vi "1A TemperatureLogger.vi"() -> ()   [LabVIEW 2011]
doc: "Elizabeth Mahon\n\nThis takes the data from the cRIO's built-in temperature sensor and saves it to a CSV file.\nPretty simple - talks to the FPGA to get the data, then sends it to a CSV file."
uses:
  <vilib>/Platform/storage/Storage.llb/usiOverwriteOptions.ctl
  <vilib>/Platform/storage/Storage.llb/usiSequenceRepresentation.ctl
  <vilib>/FPGAPlugInAG/cRIO-9113/niLvFpga_Open_cRIO-9113.vi
  <vilib>/rvi/interface/common/dynamic/niFpgaDynamicAddResources.vi
  <vilib>/Utility/error.llb/Error Cluster From Error Code.vi
  <vilib>/rvi/errors/niLvFpgaAdjustHostInterfaceError.vi
  <vilib>/FPGAPlugInAG/Dynamic/niLvFpga_Close_Dynamic.vi
  <vilib>/Platform/storage/lvStorage.llb/_openStorageWithRootAutoDetect.vi
  <vilib>/Platform/storage/lvStorage.llb/xStorage/xStorageSupp/ErrorOut.vi
  <vilib>/Platform/storage/lvStorage.llb/_createOrGetExplicitChildObject.vi
  <vilib>/Platform/storage/lvStorage.llb/_createOrGetByNameExplicitChildObject.vi
  <vilib>/Platform/storage/lvStorage.llb/_saveInt16Channel.vi
  <vilib>/Platform/storage/Storage.llb/Get Object Info.vi
  <vilib>/Platform/storage/Storage.llb/__closeStorageFromObject.vi
  <vilib>/rvi/interface/nirviOpenFPGA/nirviOpenFPGA.xnode
  FPGA Bitfiles/SailBot_FPGATarget_1ATemperatureRea_2D2CF993.lvbitx
  FPGA/1A Temperature Reader.vi
  <vilib>/rvi/interface/nirviMethod/nirviMethod.xnode
  <vilib>/rvi/interface/nirviCloseFPGA/nirviCloseFPGA.xnode
  <vilib>/Platform/storage/lvStorage.llb/xStorage/Open Data Storage/Open Data Storage.xnode
  <vilib>/Platform/storage/lvStorage.llb/xStorage/Write Data/Write Data.xnode
  <vilib>/Platform/storage/lvStorage.llb/xStorage/Close Data Storage/Close Data Storage.xnode
  <vilib>/FPGAPlugInAG/Dynamic/niLvFpga_ReadFifo_Dynamic.vi
  <vilib>/rvi/errors/niLvFpgaMergeErrorWithErrorCode.vi
panel:
  out "Temperature Data":i16[](graph)
  in  "stop":bool
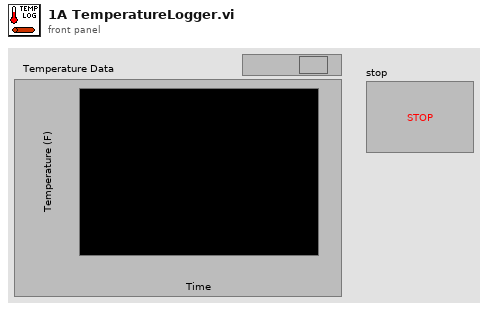
[diagram p1: front panel]
types:
  T1 = enum16{"open", "open or create", "create or replace", "create", "open (read only)"}
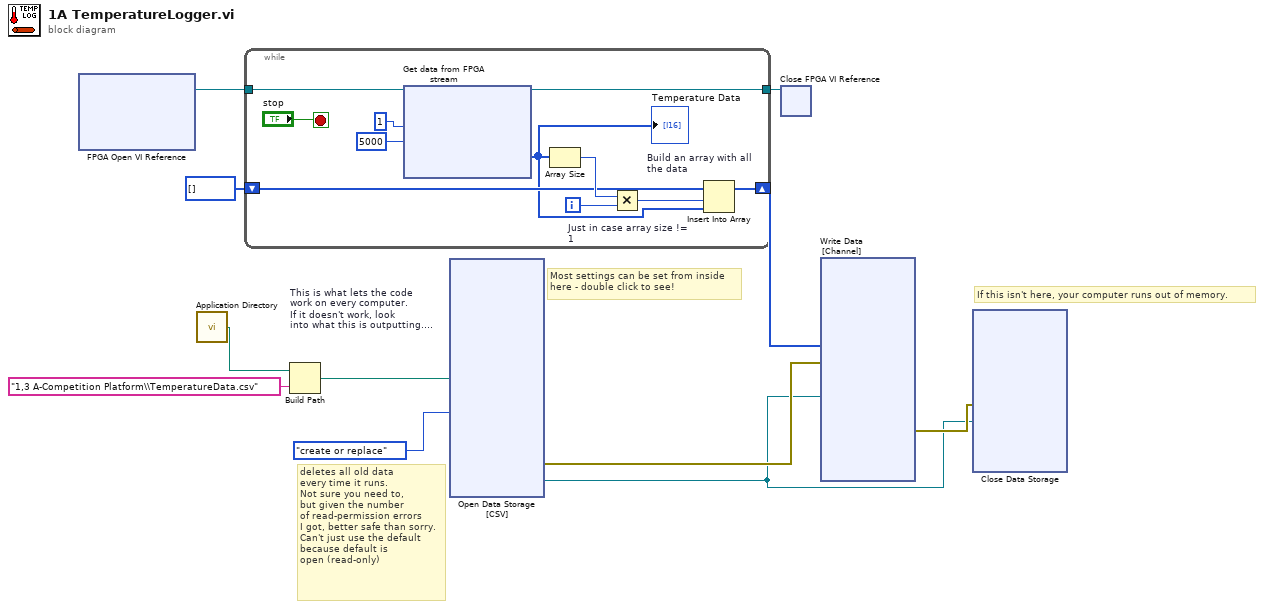
[diagram p0: block diagram]
diagram:
  # "Most settings can be set from inside\nhere - double click to see!"
  # "If this isn't here, your computer runs out of memory."
  # "deletes all old data\nevery time it runs.\nNot sure you need to,\nbut given the number\nof read-permission errors\nI got, better safe than sorry.\nCan't just use the default\nbecause default is\nopen (read-only)"
  n1 = xnode "FPGA Open VI Reference"() -> ("FPGA VI Reference Out"=w8:refnum<k20>)  [unwired: 2 in, 1 out]
  n2 = call <vilib>:"Application Directory.vi"() -> ("Application Directory"=w3:path)
  n3 = while {
    tunnel: w8 -> [w21]
    tunnel: [w20] -> w9
    shift-right: [w19] -> w6
    shift-left: i16[] [] -> [w15]
    i -> [w16]
    stop <- "stop" stop-if-true
    n4 = xnode "Get data from FPGA stream"("FPGA VI Reference In"=w21, "Number of Elements"=u32 1, "Timeout (ms)"=5000) -> ("FPGA VI Reference Out"=w20:refnum<k20>, "Data"=w12:i16[])  [unwired: 1 in, 2 out]
    "Temperature Data" <- w12
    n5 = Array Size(array=w12) -> (size(s)=w17:i32)
    n6 = Multiply "Just in case array size != 1"(x=w17, y=w16) -> (x*y=w18:i32)
    n7 = Insert Into Array "Build an array with all the data"(array=w15, index=w18, new element=w12) -> (w19:i16[])
  }
  n8 = Build Path "This is what lets the code\nwork on every computer.\nIf it doesn't work, look\ninto what this is outputting.\nCan't use default because\nthat is only for my\ncomputer!"(base path=w3, name or relative path="1,3 A-Competition Platform\\TemperatureData.csv") -> (appended path=w4:path)
  n9 = xnode "Open Data Storage\n[CSV]"("file path"=w4, "function (open:0)"=T1."create or replace") -> ("error out"=w11:errorcluster, "storage refnum (file)"=w1:refnum<k20>)  [unwired: 3 in, 1 out]
  n10 = xnode "Close FPGA VI Reference"("FPGA VI Reference In"=w9) -> ()  [unwired: 1 in, 1 out]
  n11 = xnode "Write Data\n[Channel]"("Signal"=w6, "error in"=w11, "storage refnum (file)"=w1) -> ("error out"=w10:errorcluster)  [unwired: 2 in, 2 out]
  n12 = xnode "Close Data Storage\n"("error in (no error)"=w10, "storage refnum (file)"=w1) -> ()  [unwired: 2 out]
